vi "testUnflattenPlaneAngleFromXML.vi"() -> ()   [LabVIEW 2012, in "UnitsAndXML.lvlib"]
uses:
  <userlib>/Common/UnitsAndXML/UnitsAndXML.lvlib
  <userlib>/Common/UnitsAndXML/FlattenItemWithUnitToXML/FlattenPlaneAngleToXML/PlaneAngleUnit.ctl
  <userlib>/Common/UnitsAndXML/SupportFiles/Position/Position.lvclass
  <userlib>/Common/UnitsAndXML/UnflattenItemWithUnitFromXML/UnflattenPlaneAngleFromXML/typeMethods/unflattenPlaneAngleFromXML_Array.vi
  <userlib>/Common/UnitsAndXML/UnflattenItemWithUnitFromXML/UnflattenPlaneAngleFromXML/typeMethods/unflattenPlaneAngleFromXML_Scalar.vi
panel:
  out "error out":errorcluster
  out "angles 3":dbl[unit][](array[numeric])
  out "angle 3":dbl[unit]
  out "angles 2":dbl[unit][](array[numeric])
  out "angle 2":dbl[unit]
  in  "PlaneAngleUnitInXML":T1
  in  "xmlStringArray":string="<angles>15</angles>\r\n<angles>30</angles>\r\n<angles>45</angles>\r\n<angles>60</angles>"
  in  "xmlStringScalar":string="<angle>15</angle>"
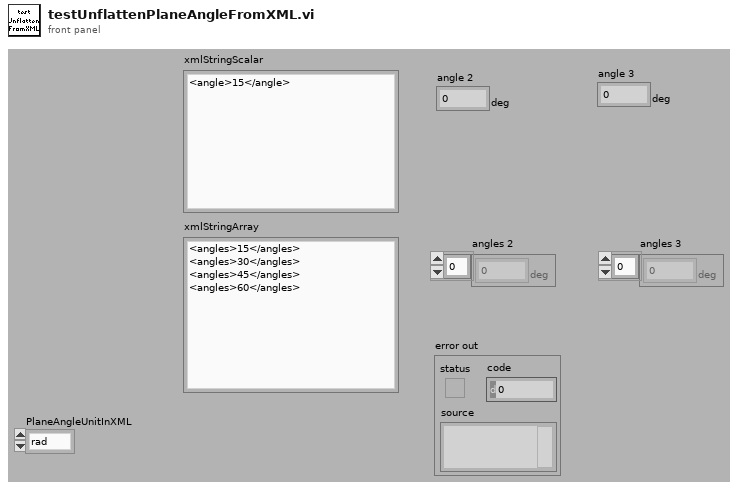
[diagram p1: front panel]
types:
  T1 = typedef "UnitsAndXML.lvlib/PlaneAngleUnit.ctl" = enum16{"rad", "deg", "'", "\""}
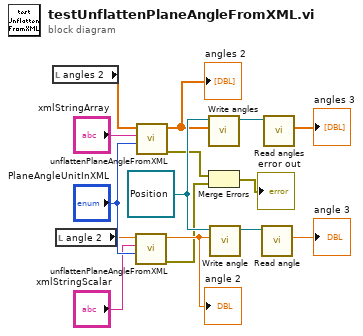
[diagram p0: block diagram]
diagram:
  w15 = refnum<class "Position.lvclass"> refnum ("Position in")
  n1 = local read "angles 2"() -> (w6:dbl[unit][])
  n2 = local read "angle 2"() -> (w7:dbl[unit])
  n3 = call-poly <userlib>:"unflattenPlaneAngleFromXML.vi"("planeAngleUnitInXML"="PlaneAngleUnitInXML", "xmlString"="xmlStringScalar", "planeAngleForType"=w7) -> ("error out"=w2:errorcluster, "planeAngle"=w11:dbl[unit])  [unwired: 7 in]
  "angle 2" <- w11
  n4 = call-poly <userlib>:"unflattenPlaneAngleFromXML.vi"("planeAngleUnitInXML"="PlaneAngleUnitInXML", "xmlString"="xmlStringArray", "planeAngleForType"=w6) -> ("error out"=w3:errorcluster, "planeAngle"=w10:dbl[unit][])  [unwired: 7 in]
  "angles 2" <- w10
  n5 = call <userlib>:"Write angles.vi"("angles"=w10, "Position in"=w15) -> ("Position out"=w14:refnum<class "Position.lvclass">)  [unwired: 8 in, 1 out]
  n6 = Merge Errors(w3, w2) -> (→"error out":errorcluster)
  n7 = call <userlib>:"Write angle.vi"("angle"=w11, "Position in"=w15) -> ("Position out"=w13:refnum<class "Position.lvclass">)  [unwired: 8 in, 1 out]
  n8 = call <userlib>:"Read angle.vi"("Position in"=w13) -> ("angle"=→"angle 3":dbl[unit])  [unwired: 8 in, 2 out]
  n9 = call <userlib>:"Read angles.vi"("Position in"=w14) -> ("angles"=→"angles 3":dbl[unit][])  [unwired: 8 in, 2 out]
